vi "Time column check.vi"(10 "Array":string[][](array[string])) -> (2 "Mistake?":bool)   [LabVIEW 2014]
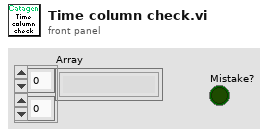
[diagram p1: front panel]
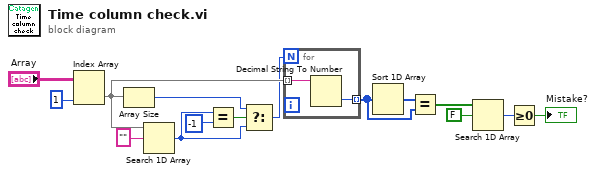
[diagram p0: block diagram]
diagram:
  n1 = Index Array(array="Array", index (col)=1 ("disabled index (col)")) -> (element=w2:string[])  [unwired: 1 in]
  n2 = Array Size(array=w2) -> (size(s)=w6:i32)
  n3 = Search 1D Array(1D array=w2, element="") -> (index of element=w7:i32)  [unwired: 1 in]
  n4 = Equal?(x=w7, y=-1) -> (x = y?=w5:bool)
  n5 = Select(t=w6, s=w5, f=w7) -> (s? t:f=w1:i32)
  n6 = for {
    N: w1 -> [_]
    tunnel: w2 -> [w17] mode=indexing
    tunnel: [w16] -> w9 mode=indexing
    n7 = Decimal String To Number(string=w17) -> (number=w16:i32)  [unwired: 2 in, 1 out]
  }
  n8 = Sort 1D Array(array=w9) -> (sorted array=w15:i32[])
  n9 = Equal?(x=w15, y=w9) -> (x = y?=w14:bool[])
  n10 = Search 1D Array(1D array=w14, element=FALSE) -> (index of element=w12:i32)  [unwired: 1 in]
  n11 = Greater Or Equal To 0?(x=w12) -> (x >= 0?=→"Mistake?":bool)
